vi "kvCanObjBufFreeAll.vi"(2 "error in (no error)":errorcluster, 3 "Channel Handle (input only)":i32) -> (0 "error out":errorcluster, 1 "Channel Handle (output only)":i32)   [LabVIEW 2022 SP3]
doc: "Releases all object buffers associated with the open handle to the CAN circuit back to the object buffer pool."
uses:
  canlib32.dll
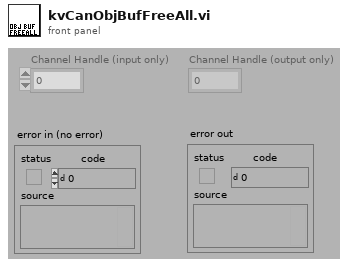
[diagram p1: front panel]
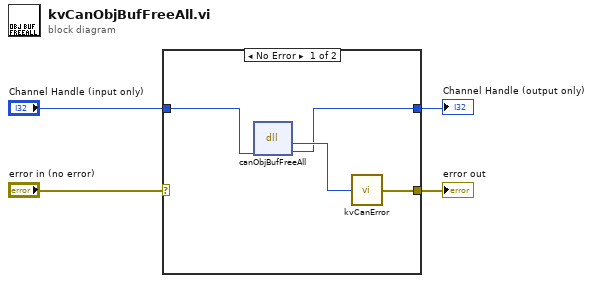
[diagram p0: block diagram]
diagram:
  n1 = case shown="No Error" "error in (no error)" {
    selector: "error in (no error)" -> [_ w9]
    tunnel: "Channel Handle (input only)" -> [w7 w10]
    tunnel: [w5 w10] -> w2
    tunnel: [w8 w9] -> w1
    frame No Error {
      n2 = dll-call lib="canlib32.dll" fn="canObjBufFreeAll"("channelHandle"=w7) -> (w6:i32, "channelHandle"=w5:i32)  [unwired: 3 in, 2 out]
      n3 = call "kvCanError.vi"("error code"=w6) -> ("error out"=w8:errorcluster)
    }
    frame Error {
    }
  }
  "error out" <- w1
  "Channel Handle (output only)" <- w2
